vi "Init Hardware.vi"(8 "error in (no error)":errorcluster, 11 "Red Pitaya Transceiver Driver in":refnum<class "Red Pitaya Transceiver Driver.lvclass">) -> (0 "error out":errorcluster, 3 "Red Pitaya Transceiver Driver out":refnum<class "Red Pitaya Transceiver Driver.lvclass">)   [LabVIEW 2016, in "Red Pitaya Transceiver Driver.lvclass"]
uses:
  Red Pitaya Transceiver Driver.lvclass
  RP Transceiver/Receiver format.ctl
  Red Pitaya Transceiver Driver.lvclass/Red Pitaya Transceiver Driver.ctl
  RP Instrument/RP Instrument.lvclass/RP Instrument.ctl
  RP Transceiver/RP Transceiver.lvclass/RP Transceiver.ctl
  Read RP Transceiver.vi
  RP Instrument/Write LED and scaler.vi
  RP Instrument/Write DDS delay.vi
  RP Transceiver/Write Receiver format.vi
  Write RP Transceiver.vi
  RP Transceiver/RP Transceiver.lvclass
  C:/github/NHMFL_Core/Libraries/Red Pitaya/RP Core/RP Instrument/RP Instrument.lvclass
  Read Spectrum Configuration.vi
  RP Instrument/Write Server address.vi
  Instruments/Instrument Driver/Instrument Driver.lvclass
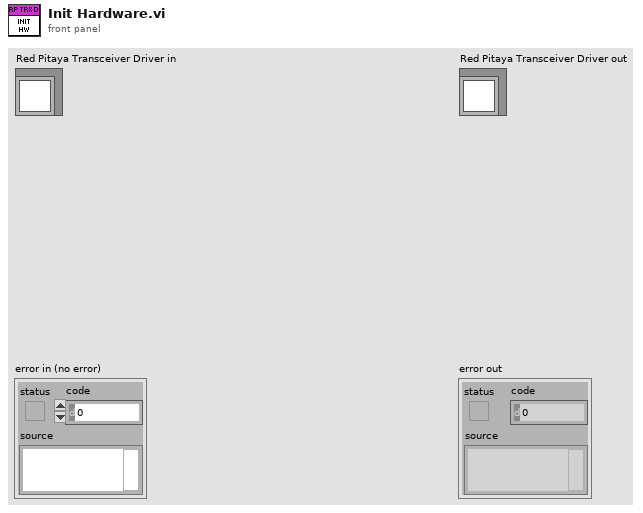
[diagram p1: front panel]
types:
  T1 = typedef "Receiver format.ctl" = enum16{"X-Y-F", "F-X-Y", "X-Y", "X"}
  T2 = typedef "Spectrum Configuration.ctl" = cluster{"Start frequency":dbl, "End frequency":dbl, "Coarse step":dbl, "Step duration":dbl, "Red Pitaya address":string, "Open plot \non start":bool, "Fine region centers":dbl[], "Regions width":dbl, "Fine step":dbl, "Pause between scans":dbl, "Clear rgs on start":bool, "Output amplitude":dbl}
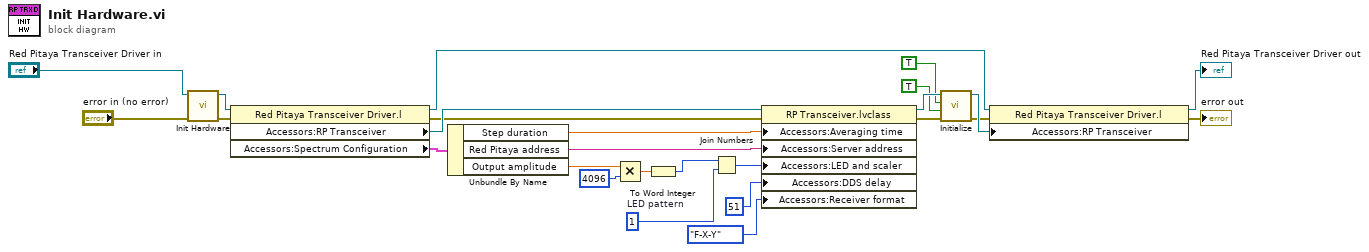
[diagram p0: block diagram]
diagram:
  w2 = i16 1  # LED pattern
  n1 = call-parent "Init Hardware.vi"("error in (no error)"="error in (no error)", "Instrument Driver in"="Red Pitaya Transceiver Driver in") -> ("error out"=w26:errorcluster, "Instrument Driver out"=w23:refnum<class "Red Pitaya Transceiver Driver.lvclass">)  [unwired: 8 in]
  n2 = property class="Red Pitaya Transceiver Driver.l"(reference=w23, error in=w26) -> (reference out=w14:refnum<class "Red Pitaya Transceiver Driver.lvclass">, error out=w20:errorcluster, "Accessors:RP Transceiver"=w22:refnum<class "RP Transceiver.lvclass">, "Accessors:Spectrum Configuration"=w21:T2)
  n3 = Unbundle By Name(w21) -> ("Step duration"=w10:dbl, "Red Pitaya address"=w9:string, "Output amplitude"=w6:dbl)
  n4 = Multiply(x=w6, y=i16 4096) -> (x*y=w4:dbl)
  n5 = To Word Integer(number=w4) -> (16bit integer=w3:i16)
  n6 = Join Numbers(hi=w3, lo=w2) -> ((hi.lo)=w1:u32)
  n7 = property class="RP Transceiver.lvclass"(reference=w22, error in=w20, "Accessors:Averaging time"=w10, "Accessors:Server address"=w9, "Accessors:LED and scaler"=w1, "Accessors:DDS delay"=u32 51 ("DDS delay"), "Accessors:Receiver format"=Receiver_format."F-X-Y" ("Receiver format")) -> (reference out=w19:refnum<class "RP Transceiver.lvclass">, error out=w16:errorcluster)
  n8 = call-dynamic "Initialize.vi"("error in (no error)"=w16, "Send \"Connect client\""=TRUE ("Send \"Connect client\""), "Reset"=TRUE, "RP Transceiver in"=w19) -> ("error out"=w12:errorcluster, "RP Transceiver out"=w15:refnum<class "RP Transceiver.lvclass">)  [unwired: 6 in]
  n9 = property class="Red Pitaya Transceiver Driver.l"(reference=w14, error in=w12, "Accessors:RP Transceiver"=w15) -> (reference out=→"Red Pitaya Transceiver Driver out":refnum<class "Red Pitaya Transceiver Driver.lvclass">, error out=→"error out":errorcluster)
